vi "setTempCommand.vi"(3 "Temperature":string) -> (0 "Command Output":string, 1 "Correct Format?":bool)   [LabVIEW 2014]
uses:
  <vilib>/regexp/Match Regular Expression.xnode
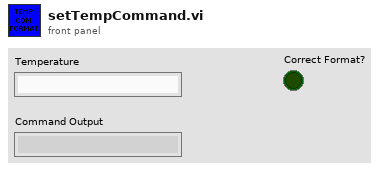
[diagram p1: front panel]
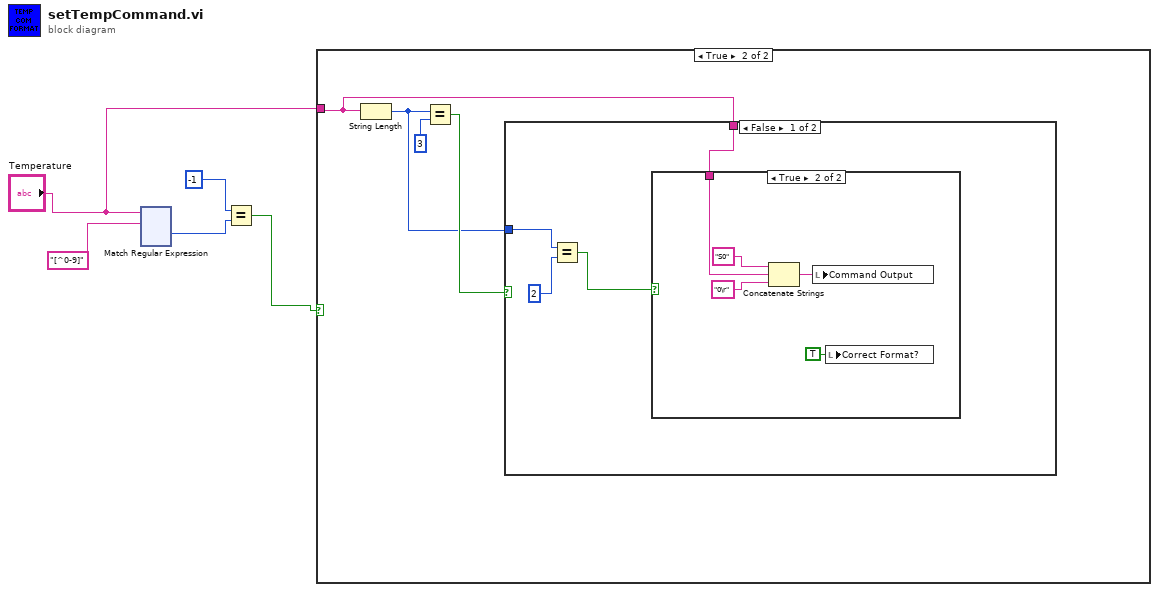
[diagram p0: block diagram]
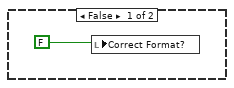
[diagram p3: hidden frame]
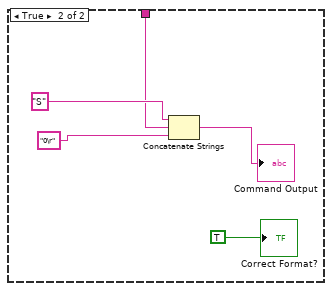
[diagram p4: hidden frame]
diagram:
  n1 = xnode "Match Regular Expression"("input string"="Temperature", "regular expression"="[^0-9]") -> ("offset past match"=w4:i32)  [unwired: 4 in, 4 out]
  n2 = Equal?(x=-1, y=w4) -> (x = y?=w2:bool)
  n3 = case shown="True" w2 {
    tunnel: "Temperature" -> [_ w6]
    frame False {
    }
    frame True {
      n4 = String Length(string=w6) -> (length=w7:i32)
      n5 = Equal?(x=w7, y=3) -> (x = y?=w9:bool)
      n6 = case shown="False" w9 {
        tunnel: w7 -> [w12 _]
        tunnel: w6 -> [w10 w20]
        frame False {
          n7 = Equal?(x=w12, y=2) -> (x = y?=w11:bool)
          n8 = case shown="True" w11 {
            tunnel: w10 -> [_ w15]
            frame False {
              n9 = local write "Correct Format?"(FALSE) -> ()
            }
            frame True {
              n10 = Concatenate Strings("S0", w15, "0\r") -> (w17:string)
              n11 = local write "Command Output"(w17) -> ()
              n12 = local write "Correct Format?"(TRUE) -> ()
            }
          }
        }
        frame True {
          n13 = Concatenate Strings("S", w20, "0\r") -> (→"Command Output":string)
          "Correct Format?" <- TRUE
        }
      }
    }
  }
